vi "Cluster Info.vi"(8 "error in (no error)":errorcluster, 11 "XNET Cluster":refnum<k21>) -> (0 "error out":errorcluster)   [LabVIEW 2009, in "NI-XNET Custom Device.lvlib"]
uses:
  NI-XNET Custom Device.lvlib
  Program Files/National Instruments/LabVIEW 2009/examples/nixnet/examples.llb/NI-XNET Example Control - FlexRay Cluster Advanced.ctl
  Program Files/National Instruments/LabVIEW 2009/resource/objmgr/xnet.rc
panel:
  in  "Done":bool
  in  "FlexRay Advanced Cluster 2":T1={"Action Point Offset"=0, "CAS Rx Low Max"=0, "Cluster Drift Damping"=0, "Cold Start Attempts"=0, "Dynamic Slot Idle Phase"=0, "Listen Noise"=0, "Macro Per Cycle"=0, "Without Clock Correction Fatal"=0, "Max Without Clock Correction Passive"=0, "Minislot Action Point Offset"=0, "Minislot"=0, "Network Management Vector Length"=0, "NIT"=0, "Number Of Minislots"=0, "Offset Correction Start"=0, "Payload Length Dynamic Maximum"=0, "Static Slot"=0, "Symbol Window"=0, "Sync Node Max"=0, "TSS Transmitter"=0, "Wakeup Symbol Rx Idle"=0, "Wakeup Symbol Rx Low"=0, "Wakeup Symbol Rx Window"=0, "Wakeup Symbol Tx Idle"=0, "Wakeup Symbol Tx Low"=0, "Cycle Time"=5000, "Number of Static Slots"=75, "Static Frame Payload Length"=8, "Baud Rate"=10000000, "Channels"=1, "Cluster Name"="FlexRayAdvancedCluster", "Comment"="", "Use Symbol Window"=FALSE} {"Channels" items=["A only"=1, "B only"=2, "A and B"=3]; "Baud Rate" items=["10 Mbps"=10000000, "5 Mbps"=5000000, "2.5 Mbps"=2500000]; "Static Frame Payload Length" max=254 step=2 format="%.0f Byte(s)"; "Number of Static Slots" min=2 max=1023 step=1; "Cycle Time" min=10 max=16000 step=1 format="%.0f µs"}
  out "FlexRay Advanced Cluster":T1={"Action Point Offset"=0, "CAS Rx Low Max"=0, "Cluster Drift Damping"=0, "Cold Start Attempts"=0, "Dynamic Slot Idle Phase"=0, "Listen Noise"=0, "Macro Per Cycle"=0, "Without Clock Correction Fatal"=0, "Max Without Clock Correction Passive"=0, "Minislot Action Point Offset"=0, "Minislot"=0, "Network Management Vector Length"=0, "NIT"=0, "Number Of Minislots"=0, "Offset Correction Start"=0, "Payload Length Dynamic Maximum"=0, "Static Slot"=0, "Symbol Window"=0, "Sync Node Max"=0, "TSS Transmitter"=0, "Wakeup Symbol Rx Idle"=0, "Wakeup Symbol Rx Low"=0, "Wakeup Symbol Rx Window"=0, "Wakeup Symbol Tx Idle"=0, "Wakeup Symbol Tx Low"=0, "Cycle Time"=5000, "Number of Static Slots"=75, "Static Frame Payload Length"=8, "Baud Rate"=10000000, "Channels"=1, "Cluster Name"="FlexRayAdvancedCluster", "Comment"="", "Use Symbol Window"=FALSE} {"Channels" items=["A only"=1, "B only"=2, "A and B"=3]; "Baud Rate" items=["10 Mbps"=10000000, "5 Mbps"=5000000, "2.5 Mbps"=2500000]; "Static Frame Payload Length" max=254 step=2 format="%.0f Byte(s)"; "Number of Static Slots" min=2 max=1023 step=1; "Cycle Time" min=10 max=16000 step=1 format="%.0f µs"}
  # "Static Segment"
  # "Dynamic Segment"
  # "Schedule"
  # "Others"
  # "General"
  # "Wakeup"
  # "Static Segment"
  # "Dynamic Segment"
  # "Schedule"
  # "Others"
  # "General"
  # "Wakeup"
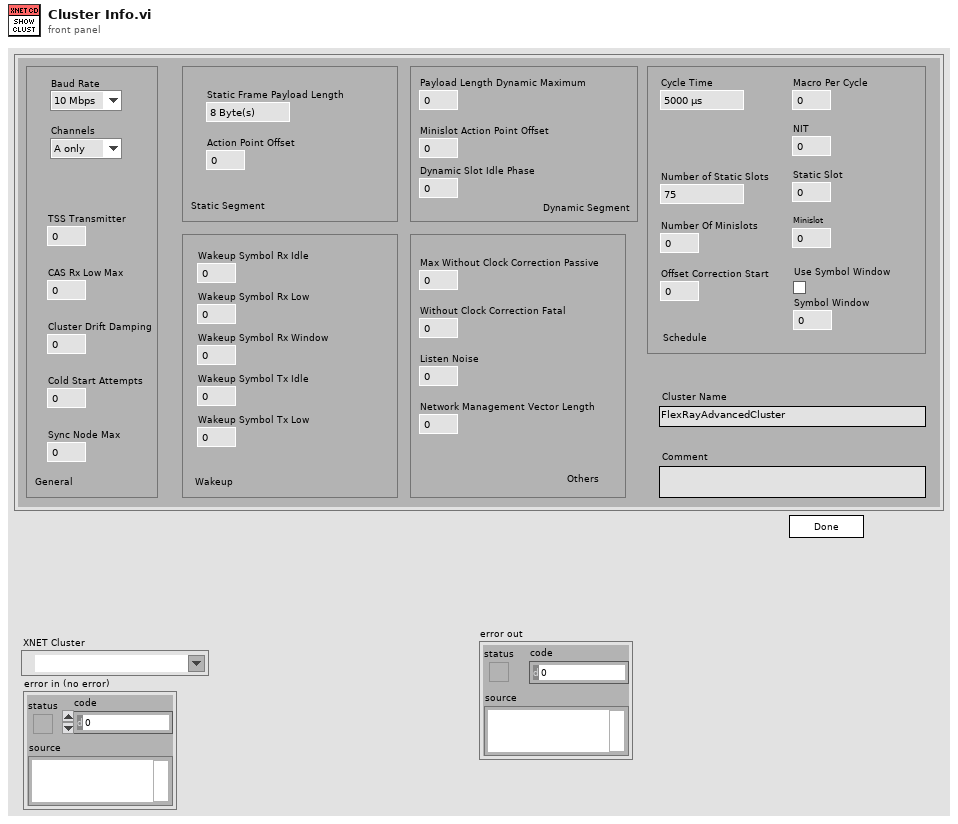
[diagram p1: front panel]
types:
  T1 = typedef "NI-XNET Example Control - FlexRay Cluster Advanced.ctl" = cluster{"Action Point Offset":u32, "CAS Rx Low Max":u32, "Cluster Drift Damping":u32, "Cold Start Attempts":u32, "Dynamic Slot Idle Phase":u32, "Listen Noise":u32, "Macro Per Cycle":u32, "Without Clock Correction Fatal":u32, "Max Without Clock Correction Passive":u32, "Minislot Action Point Offset":u32, "Minislot":u32, "Network Management Vector Length":u32, "NIT":u32, "Number Of Minislots":u32, "Offset Correction Start":u32, "Payload Length Dynamic Maximum":u32, "Static Slot":u32, "Symbol Window":u32, "Sync Node Max":u32, "TSS Transmitter":u32, "Wakeup Symbol Rx Idle":u32, "Wakeup Symbol Rx Low":u32, "Wakeup Symbol Rx Window":u32, "Wakeup Symbol Tx Idle":u32, "Wakeup Symbol Tx Low":u32, "Cycle Time":u32, "Number of Static Slots":u32, "Static Frame Payload Length":u32, "Baud Rate":u32, "Channels":u32, "Cluster Name":string, "Comment":string, "Use Symbol Window":bool}
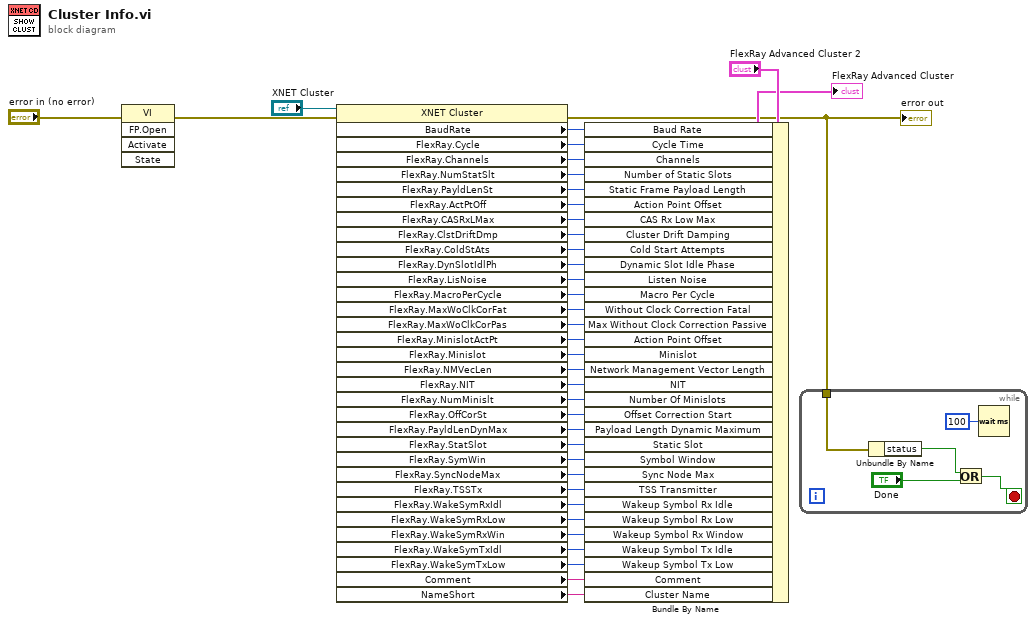
[diagram p0: block diagram]
diagram:
  n1 = invoke class="VI" method="FP.Open"(error in="error in (no error)") -> (error out=w2:errorcluster)  [unwired: 4 in, 4 out]
  n2 = property class="XNET Cluster"(reference="XNET Cluster", error in=w2) -> (error out=w4:errorcluster, "BaudRate"=w35:u32, "FlexRay.Cycle"=w34:u32, "FlexRay.Channels"=w33:u32, "FlexRay.NumStatSlt"=w32:u32, "FlexRay.PayldLenSt"=w31:u32, "FlexRay.ActPtOff"=w30:u32, "FlexRay.CASRxLMax"=w29:u32, "FlexRay.ClstDriftDmp"=w28:u32, "FlexRay.ColdStAts"=w27:u32, "FlexRay.DynSlotIdlPh"=w26:u32, "FlexRay.LisNoise"=w25:u32, "FlexRay.MacroPerCycle"=w24:u32, "FlexRay.MaxWoClkCorFat"=w23:u32, "FlexRay.MaxWoClkCorPas"=w22:u32, "FlexRay.MinislotActPt"=w21:u32, "FlexRay.Minislot"=w20:u32, "FlexRay.NMVecLen"=w19:u32, "FlexRay.NIT"=w18:u32, "FlexRay.NumMinislt"=w17:u32, "FlexRay.OffCorSt"=w16:u32, "FlexRay.PayldLenDynMax"=w15:u32, "FlexRay.StatSlot"=w14:u32, "FlexRay.SymWin"=w13:u32, "FlexRay.SyncNodeMax"=w12:u32, "FlexRay.TSSTx"=w11:u32, "FlexRay.WakeSymRxIdl"=w10:u32, "FlexRay.WakeSymRxLow"=w9:u32, "FlexRay.WakeSymRxWin"=w8:u32, "FlexRay.WakeSymTxIdl"=w7:u32, "FlexRay.WakeSymTxLow"=w6:u32, "Comment"=w5:string, "NameShort"=w1:string)  [unwired: 1 out]
  "error out" <- w4
  n3 = Bundle By Name(cluster="FlexRay Advanced Cluster 2", "Baud Rate"=w35, "Cycle Time"=w34, "Channels"=w33, "Number of Static Slots"=w32, "Static Frame Payload Length"=w31, "Action Point Offset"=w30, "CAS Rx Low Max"=w29, "Cluster Drift Damping"=w28, "Cold Start Attempts"=w27, "Dynamic Slot Idle Phase"=w26, "Listen Noise"=w25, "Macro Per Cycle"=w24, "Without Clock Correction Fatal"=w23, "Max Without Clock Correction Passive"=w22, "Action Point Offset"=w21, "Minislot"=w20, "Network Management Vector Length"=w19, "NIT"=w18, "Number Of Minislots"=w17, "Offset Correction Start"=w16, "Payload Length Dynamic Maximum"=w15, "Static Slot"=w14, "Symbol Window"=w13, "Sync Node Max"=w12, "TSS Transmitter"=w11, "Wakeup Symbol Rx Idle"=w10, "Wakeup Symbol Rx Low"=w9, "Wakeup Symbol Rx Window"=w8, "Wakeup Symbol Tx Idle"=w7, "Wakeup Symbol Tx Low"=w6, "Comment"=w5, "Cluster Name"=w1) -> (→"FlexRay Advanced Cluster":T1)
  n4 = while {
    tunnel: w4 -> [w43]
    stop <- w42 stop-if-true
    n5 = Unbundle By Name(w43) -> ("status"=w41:bool)
    n6 = Or(x=w41, y="Done") -> (x .or. y?=w42:bool)
    n7 = Wait (ms)(milliseconds to wait=u32 100) -> ()  [unwired: 1 out]
  }
